vi "PicoScope3000aExampleAWG.vi"() -> ()   [LabVIEW 2010]
uses:
  PS3000a.dll
panel:
  in  "error in (no error)":errorcluster
  out "USB 3.0 device on non-USB 3.0 Port":bool=TRUE
  out "USB Powered":bool=TRUE
  out "error out":errorcluster
  in  "Arbitrary Waveform Settings":T1 {"Index Mode" items=["Single", "Dual", "Quad"]}
  in  "General AWG Settings":T2={"Peak-to-Peak Voltage (microvolts)"=2000000, "Offset Voltage (microvolts)"=0, "Wave Type"=0, "Sweep Type"=0, "Shots"=0, "Sweeps"=0, "Trigger Type"=0, "Trigger Source"=0, "Ext. Threshold (ADC count)"=0, "White Noise/PRBS"=0} {"White Noise/PRBS" items=["Normal", "White Noise", "PRBS"]; "Trigger Source" items=["None", "Scope Trigger", "Aux. In", "Ext. In", "Software Trigger"]; "Trigger Type" items=["Rising", "Falling", "Gate High", "Gate Low"]; "Sweep Type" items=["Up", "Down", "Up-Down", "Down-Up"]; "Wave Type" items=["Sine"=0, "Square"=1, "Triangle"=2, "Ramp Up"=3, "Ramp Down"=4, "DC"=8, "Arbitrary"=6]}
  in  "Standard Waveform Settings":T3={"Start Frequency"=1000.0, "Stop Frequency"=1000.0, "Increment"=0.0, "Dwell Time (seconds)"=0.0} {"Stop Frequency" min=0.03 max=1000000.0 format="%#_6p"; "Start Frequency" min=0.03 max=1000000.0 format="%#_6p"}
  in  "Stop S/W \nTrigger":bool
  in  "Apply Settings":bool
  in  "Stop VI":bool
  in  "Software \nTrigger":bool
  out "Arbitrary\nWaveform Graph":i16[](graph)
  # "If Software trigger is selected, press the 'Stop S/W Trigger'\nbutton prior to selecting 'Apply Settings' or 'Stop VI'."
  # "Sweep is disabled when 'Increment' or 'Dwell Time' is set to 0, then 'Start frequency' is used"
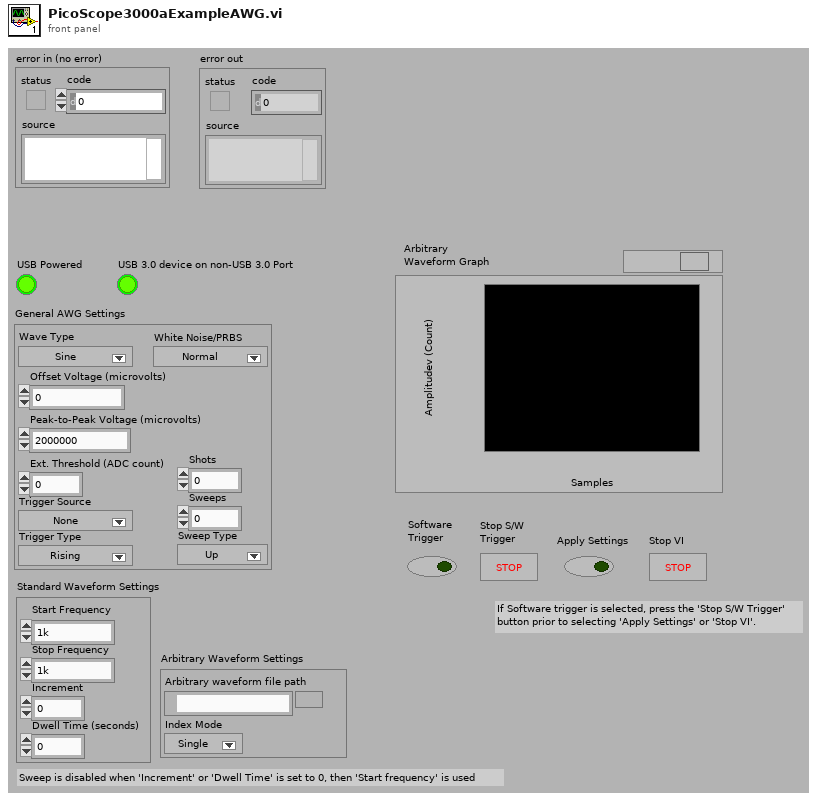
[diagram p1: front panel]
types:
  T1 = cluster{"Arbirary waveform file path":path, "Index Mode":u32}
  T2 = cluster{"Peak-to-Peak Voltage (microvolts)":u32, "Offset Voltage (microvolts)":i32, "Wave Type":i16, "Sweep Type":i32, "Shots":u32, "Sweeps":u32, "Trigger Type":i32, "Trigger Source":i32, "Ext. Threshold (ADC count)":i16, "White Noise/PRBS":u32}
  T3 = cluster{"Start Frequency":dbl, "Stop Frequency":dbl, "Increment":dbl, "Dwell Time (seconds)":dbl}
  T4 = cluster{"Driver Version":string, "USB Version":string, "Hardware":string, "Variant":string, "Batch and Serial":string, "Cal Date":string, "Kernel Version":string, "Digital HW Version":string, "Analogue HW Version":string, "MSO":bool, "Number of channels":i16}
  T5 = cluster{"status":bool, "code":u32, "source":string}
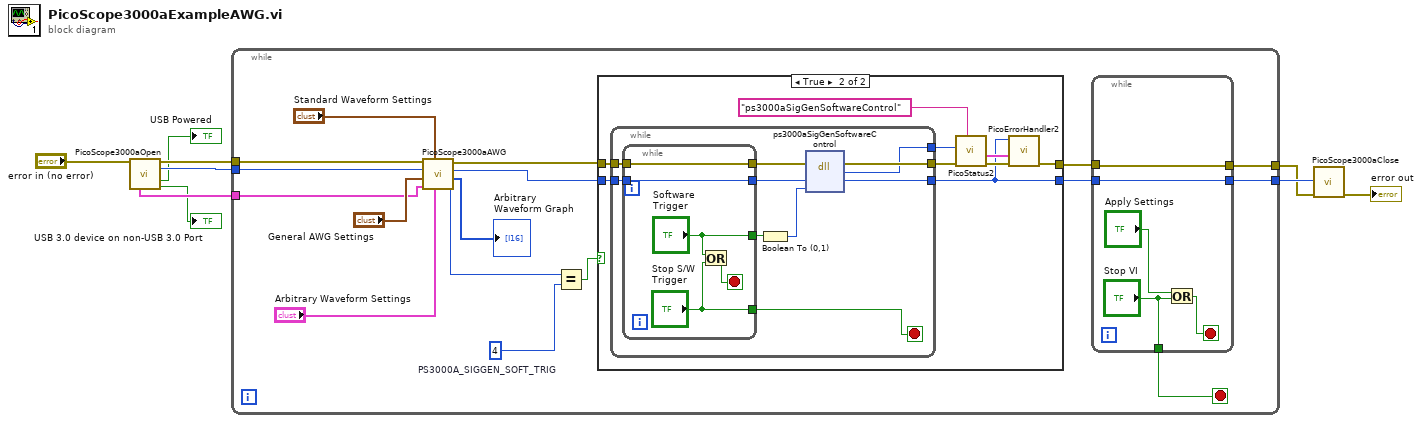
[diagram p0: block diagram]
diagram:
  n1 = call "PicoScope3000aOpen.vi"("error in (no error)"="error in (no error)") -> ("error out"=w8:errorcluster, "handle"=w9:i16, "USB Powered"=→"USB Powered":bool, "Device Info"=w6:T4, "USB 3.0 device on non-USB 3.0 Port"=→"USB 3.0 device on non-USB 3.0 Port":bool)  [unwired: 8 in, 2 out]
  n2 = while {
    tunnel: w9 -> [w25]
    tunnel: w8 -> [w24]
    tunnel: [w18] -> w7
    tunnel: w6 -> [w12]
    tunnel: [w10] -> w2
    stop <- w16 stop-if-true
    w23 = 4  # PS3000A_SIGGEN_SOFT_TRIG
    n3 = call "PicoScope3000aAWG.vi"("Arbitrary Waveform Settings"="Arbitrary Waveform Settings", "Standard Waveform Settings"="Standard Waveform Settings", "Device Info"=w12, "General AWG Settings"="General AWG Settings", "Handle In"=w25, "error in"=w24) -> ("Trigger Source Out"=w19:i32, "Arbitrary\nWaveform Graph"=→"Arbitrary\nWaveform Graph":i16[], "Handle Out"=w20:i16, "error out"=w21:errorcluster)  [unwired: 2 in]
    n4 = Equal?(x=w19, y=w23) -> (x = y?=w22:bool)
    n5 = case shown="True" w22 {
      tunnel: w21 -> [w32 w42]
      tunnel: [w33 w34] -> w17
      tunnel: w20 -> [w33 w41]
      tunnel: [w32 w35] -> w11
      frame False {
      }
      frame True {
        n6 = while {
          tunnel: w42 -> [w51]
          tunnel: w41 -> [w50]
          tunnel: [w48] -> w34
          tunnel: [w44] -> w39
          tunnel: [w43] -> w38
          stop <- w45 stop-if-true
          n7 = while {
            tunnel: [w57] -> w52
            tunnel: w51 -> [w57]
            tunnel: ["Software \nTrigger"] -> w47
            tunnel: w50 -> [w56]
            tunnel: [w56] -> w49
            tunnel: ["Stop S/W \nTrigger"] -> w45
            stop <- w53 stop-if-true
            n8 = Or(x="Software \nTrigger", y="Stop S/W \nTrigger") -> (x .or. y?=w53:bool)
          }
          n9 = Boolean To (0,1)(Boolean=w47) -> (0, 1=w46:i16)
          n10 = dll-call lib="ps3000a.dll" fn="ps3000aSigGenSoftwareControl"(error in=w52, "handle"=w49, "state"=w46) -> (error out=w44:errorcluster, "PICO_STATUS"=w43:u32, "handle"=w48:i16)  [unwired: 3 in, 1 out]
        }
        n11 = call "PicoStatus2.vi"("PICO source"="ps3000aSigGenSoftwareControl" ("source"), "Error in"=w39, "PICO STATUS"=w38) -> ("error out"=w37:errorcluster, "PICO_STATUS out"=w36:T5)  [unwired: 5 in]
        n12 = call "PicoErrorHandler2.vi"("error in (no error)"=w37, "PICO_STATUS in"=w36, "handle In"=w34) -> ("error out"=w35:errorcluster)  [unwired: 8 in]
      }
    }
    n13 = while {
      tunnel: ["Stop VI"] -> w16
      tunnel: [w31] -> w18
      tunnel: w17 -> [w31]
      tunnel: w11 -> [w27]
      tunnel: [w27] -> w10
      stop <- w30 stop-if-true
      n14 = Or(x="Apply Settings", y="Stop VI") -> (x .or. y?=w30:bool)
    }
  }
  n15 = call "PicoScope3000aClose.vi"("error in (no error)"=w2, "handle in"=w7) -> ("error out"=→"error out":errorcluster)  [unwired: 8 in, 1 out]
